vi "LabVIEW Time to TAI Time.vi"(5 "LabVIEW Time (s)":timestamp) -> (2 "TAI Time (ns)":i64)   [LabVIEW 2021, in "Time_CIF_U.lvlib"]
doc: "Convert LabVIEW time into TAI time by changing the epoch. TAI time is used as the basis of UTC and is GPS time. It is UTC without leap seconds."
uses:
  Time_CIF_U.lvlib
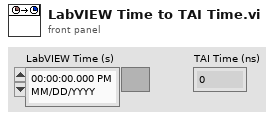
[diagram p1: front panel]
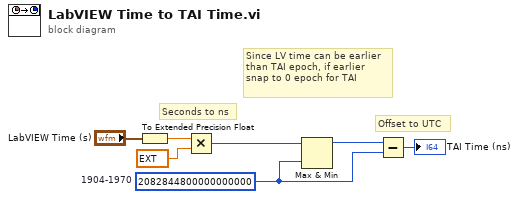
[diagram p0: block diagram]
diagram:
  w1 = i64 2082844800000000000  # 1904-1970
  # "Since LV time can be earlier than TAI epoch, if earlier snap to 0 epoch for TAI"
  # "Seconds to ns"
  # "Offset to UTC"
  n1 = To Extended Precision Float(1:"LabVIEW Time (s)") -> (0:w6:ext)
  n2 = Multiply(x=w6, y=ext 1000000000.0) -> (x*y=w3:i64)
  n3 = Max & Min(x=w3, y=w1) -> (max(x,y)=w2:i64)  [unwired: 1 out]
  n4 = Subtract(x=w2, y=w1) -> (x-y=→"TAI Time (ns)":i64)
